vi "HandleStop.vi"(8 "error in (no error)":errorcluster, 11 "Application Data":T1) -> (0 "error out":errorcluster)   [LabVIEW 2019]
uses:
  Typedefs/#cluster_ApplicationData.ctl
  Typedefs/Acquisition Thread/#cluster_AcqQueueData.ctl
  Typedefs/Acquisition Thread/#enum_AcquisitionTask.ctl
  Typedefs/Saving Thread/#cluster_SavingQueueData.ctl
  Typedefs/Saving Thread/#enum_SavingTask.ctl
  <vilib>/ActorFramework/Message Enqueuer/Message Enqueuer.lvclass
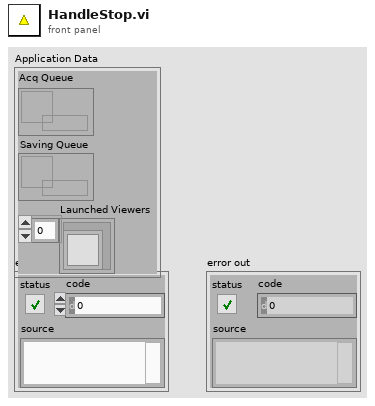
[diagram p1: front panel]
types:
  T1 = typedef "#cluster_ApplicationData.ctl" = cluster{"Acq Queue":refnum<queue>, "Saving Queue":refnum<queue>, "Launched Viewers":refnum<class "Message Enqueuer.lvclass">[]}
  T2 = typedef "#cluster_SavingQueueData.ctl" = cluster{"Task":T3, "Data":variant}
  T3 = typedef "#enum_SavingTask.ctl" = enum16{"Set directory", "Save", "Stop", "Close"}
  T4 = typedef "#cluster_AcqQueueData.ctl" = cluster{"Task":T5, "Data":variant}
  T5 = typedef "#enum_AcquisitionTask.ctl" = enum16{"Init", "Start", "Finish", "Close"}
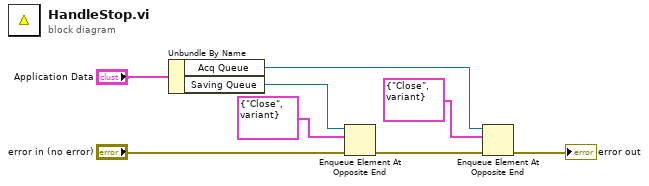
[diagram p0: block diagram]
diagram:
  n1 = Unbundle By Name("Application Data") -> ("Acq Queue"=w4:refnum<queue>, "Saving Queue"=w3:refnum<queue>)
  n2 = Enqueue Element At Opposite End(queue=w3, element=T2 {"Task"=enum."Close", "Data"=variant}, error in (no error)="error in (no error)") -> (error out=w7:errorcluster)  [unwired: 1 in, 2 out]
  n3 = Enqueue Element At Opposite End(queue=w4, element=T4 {"Task"=enum."Close", "Data"=variant}, error in (no error)=w7) -> (error out=→"error out":errorcluster)  [unwired: 1 in, 2 out]
